vi "openiscotest.vi"() -> ()   [LabVIEW 2014]
panel:
  out "添加的路径":path
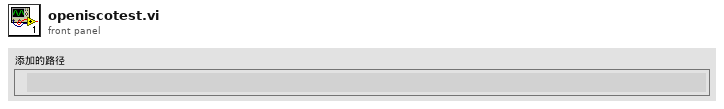
[diagram p1: front panel]
types:
  T1 = enum32{"Invalid", "Standard", "Closed", "Hidden", "Minimized", "Maximized"}
  T2 = enum32{"Bad", "Idle", "Run top level", "Running"}
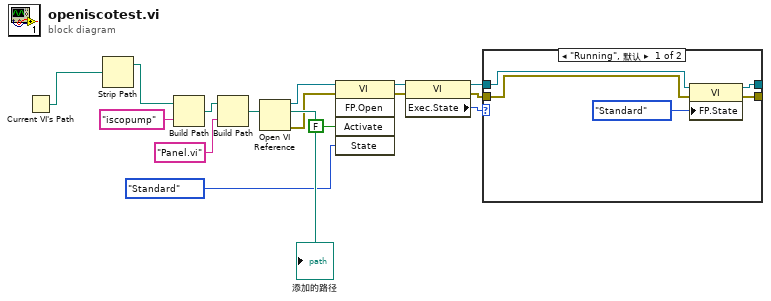
[diagram p0: block diagram]
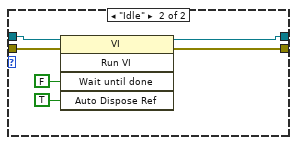
[diagram p2: hidden frame]
diagram:
  n1 = Current VI's Path ("当前VI路径")() -> (path=w2:path)
  n2 = Strip Path(path=w2) -> (stripped path=w1:path)  [unwired: 1 out]
  n3 = Build Path(base path=w1, name or relative path="iscopump" ("名称或相对路径")) -> (appended path=w15:path)
  n4 = Build Path(base path=w15, name or relative path="Panel.vi" ("名称或相对路径")) -> (appended path=w13:path)
  "添加的路径" <- w13
  n5 = Open VI Reference(vi path=w13) -> (vi reference=w12:refnum<vi>, error out=w11:errorcluster)  [unwired: 5 in]
  n6 = invoke class="VI" method="FP.Open"(reference=w12, error in=w11, "Activate"=FALSE ("激活？"), "State"=T1."Standard" ("状态")) -> (reference out=w8:refnum<vi>, error out=w7:errorcluster)  [unwired: 1 in, 3 out]
  n7 = property class="VI"(reference=w8, error in=w7) -> (reference out=w5:refnum<vi>, error out=w4:errorcluster, "Exec.State"=w6:T2)
  n8 = case shown="\"Running\", 默认" w6 {
    tunnel: [w16 w26] -> _
    tunnel: [w18 w25] -> _
    tunnel: w5 -> [w19 w22]
    tunnel: w4 -> [w17 w21]
    frame "Running", Default {
      n9 = property class="VI"(reference=w19, error in=w17, "FP.State"=T1."Standard" ("前面板窗口:状态")) -> (reference out=w18:refnum<vi>, error out=w16:errorcluster)
    }
    frame "Idle" {
      n10 = invoke class="VI" method="Run VI"(reference=w22, error in=w21, "Wait until done"=FALSE ("结束前等待"), "Auto Dispose Ref"=TRUE ("自动销毁引用")) -> (reference out=w25:refnum<vi>, error out=w26:errorcluster)  [unwired: 1 in, 3 out]
    }
  }
